vi "Sound XML File Creator.vi"() -> ()   [LabVIEW 2010]
doc: "Creates an XML file that contains data for several types of sound. \n\nThis XML file will be read by Sound Demo.lvclass:Execute.vi to obtain the sounds that will be played by the Sound Player Demo."
uses:
  Silence/Silence.lvclass
  Fade/Fade.lvclass
  Recorded Sound/Recorded Sound.lvclass
  <vilib>/Utility/xml.llb/Write to XML File(string).vi
  Aggregate Sound/Aggregate Sound.lvclass
panel:
  out "error out":errorcluster
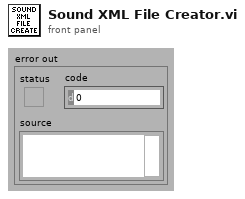
[diagram p1: front panel]
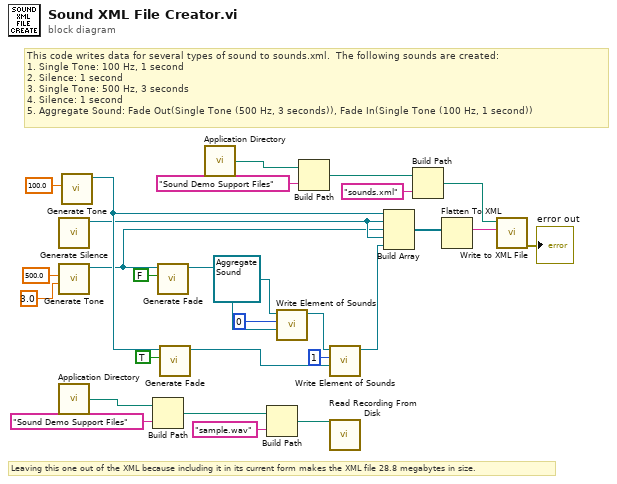
[diagram p0: block diagram]
diagram:
  # "This code writes data for several types of sound to sounds.xml.  The following sounds are created:\n1. Single Tone: 100 Hz, 1 second\n2. Silence: 1 second\n3. Single Tone: 500 Hz, 3 seconds\n4. Silence: 1 second\n5. Aggregate Sound: Fade Out(Single Tone (500 Hz, 3 seconds)), Fade In(Single Tone (100 Hz, 1 second))"
  # "Leaving this one out of the XML because including it in its current form makes the XML file 28.8 megabytes in size."
  n1 = call "Generate Silence.vi"() -> ("Silence out"=w7:refnum<class "Silence.lvclass">)  [unwired: 11 in]
  n2 = call "Generate Tone.vi"("Duration (1 second)"=3.0, "Frequency (500 Hz)"=500.0 ("Frequency")) -> ("Single Tone out"=w6:refnum<class "Single Tone.lvclass">)  [unwired: 9 in]
  n3 = call <vilib>:"Application Directory.vi"() -> ("Application Directory"=w2:path)
  n4 = call "Generate Tone.vi"("Frequency (500 Hz)"=100.0 ("Frequency")) -> ("Single Tone out"=w14:refnum<class "Single Tone.lvclass">)  [unwired: 10 in]
  n5 = Build Path(base path=w2, name or relative path="Sound Demo Support Files") -> (appended path=w4:path)
  n6 = call "Generate Fade.vi"("Fade in? (True)"=FALSE, "Original Sound"=w6) -> ("Fade"=w12:refnum<class "Fade.lvclass">)  [unwired: 9 in]
  n7 = call "Generate Fade.vi"("Fade in? (True)"=TRUE, "Original Sound"=w14) -> ("Fade"=w11:refnum<class "Fade.lvclass">)  [unwired: 9 in]
  n8 = call <vilib>:"Application Directory.vi"() -> ("Application Directory"=w23:path)
  n9 = Build Path(base path=w4, name or relative path="sample.wav") -> (appended path=w1:path)
  n10 = call "Write Element of Sounds.vi"("Sound.lvclass"=w12, "index"=0, "Aggregate Sound in"=refnum<class "Aggregate Sound.lvclass"> refnum) -> ("Aggregate Sound out"=w10:refnum<class "Aggregate Sound.lvclass">)  [unwired: 8 in]
  n11 = Build Path(base path=w23, name or relative path="Sound Demo Support Files") -> (appended path=w21:path)
  n12 = call "Write Element of Sounds.vi"("Sound.lvclass"=w11, "index"=1, "Aggregate Sound in"=w10) -> ("Aggregate Sound out"=w8:refnum<class "Aggregate Sound.lvclass">)  [unwired: 8 in]
  n13 = call "Read Recording From Disk.vi"("File Path"=w1) -> ()  [unwired: 9 in, 2 out]
  n14 = Build Array(w14, w7, w6, w7, w8) -> (w24:refnum<class>[])
  n15 = Build Path(base path=w21, name or relative path="sounds.xml") -> (appended path=w17:path)
  n16 = Flatten To XML(anything=w24) -> (xml string=w18:string)
  n17 = call-poly <vilib>:"Write to XML File.vi"("XML Input"=w18, "XML File Path"=w17) -> ("error out"=→"error out":errorcluster)  [unwired: 7 in, 2 out]
